vi "CreateGraphRightKeyMenu.vi"(4 "isFloatXY":T1, 6 "isShowYvalue":T1, 8 "Language":refnum<vi>, 9 "Coords":T3, 10 "MenuRef":refnum<k9>, 11 "XYGraph输入":refnum<vi>) -> ()   [LabVIEW 2015]
uses:
  <vilib>/Utility/miscctls.llb/LVPoint32TypeDef.ctl
  Ctrls/YesOrNo.ctl
panel:
  in  "WhereIsMouse":T2(ring)
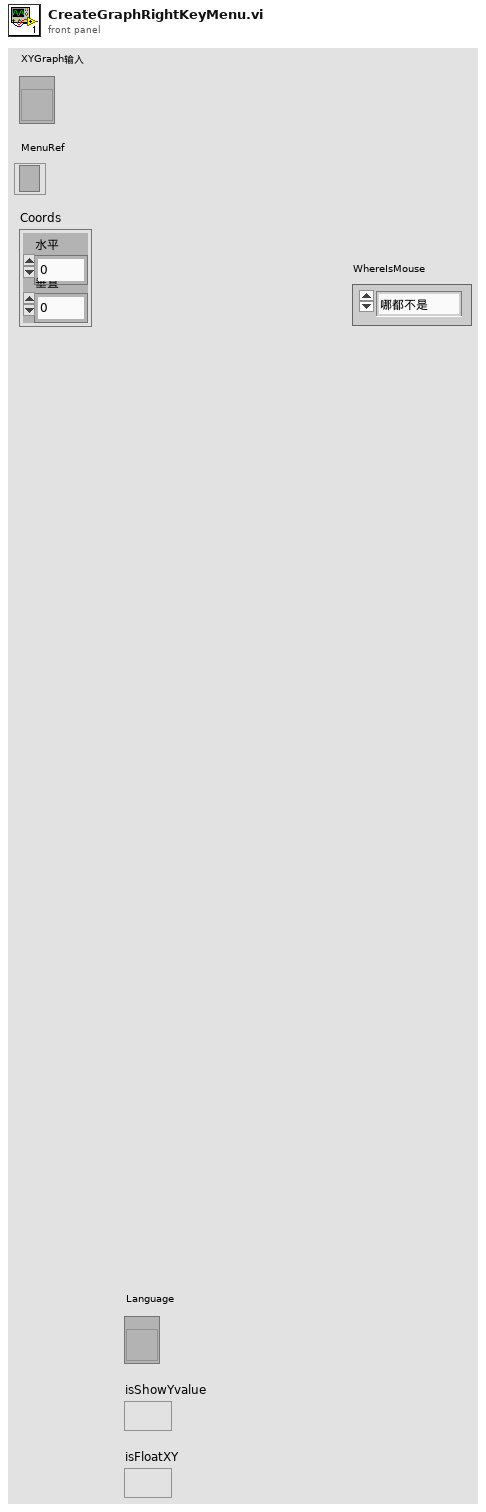
[diagram p1: front panel]
types:
  T1 = typedef "YesOrNo.ctl" = bool
  T2 = enum16{"哪都不是", "在曲线上", "在X轴上", "在单Y轴上", "在绘图区域但非曲线上", "在绘图区域上方", "在图例上"}
  T3 = typedef "LVPoint32TypeDef.ctl" = cluster{"Horizontal":i32, "Vertical":i32}
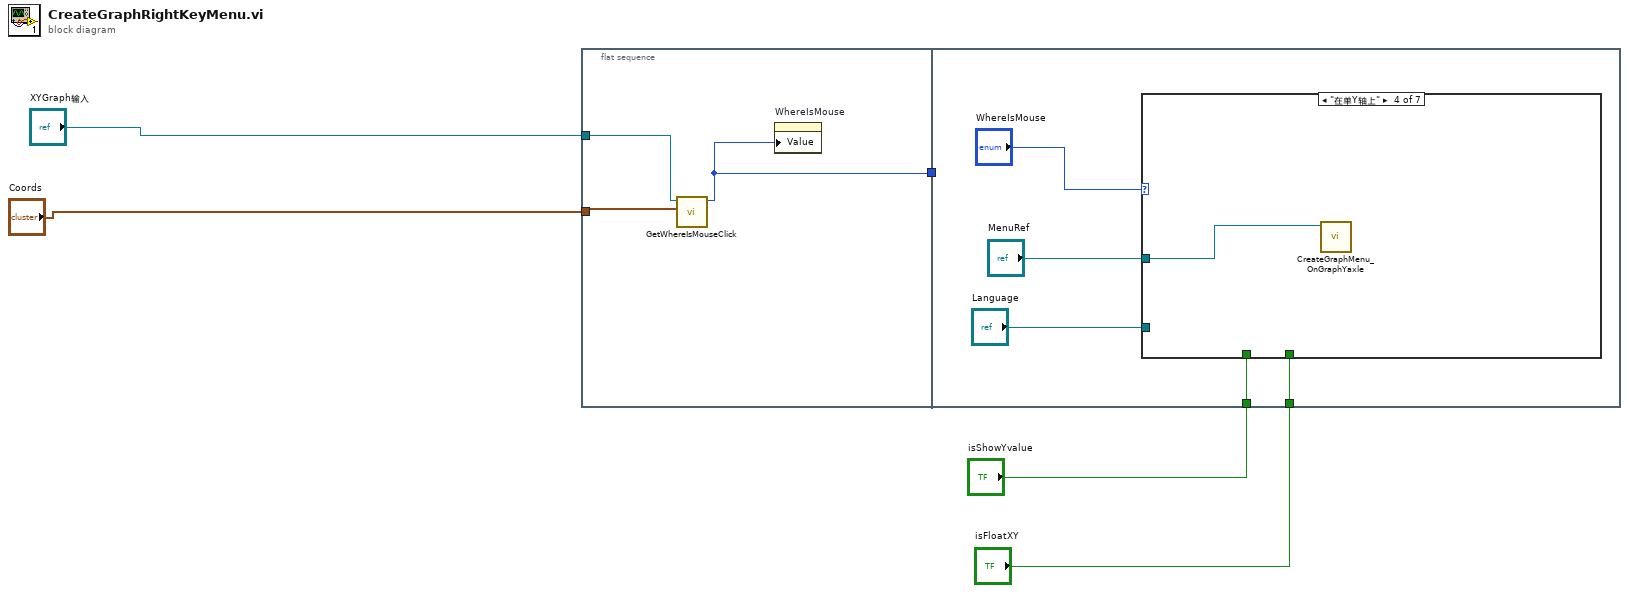
[diagram p0: block diagram]
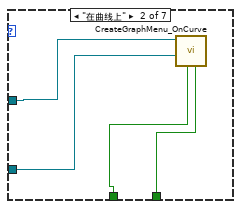
[diagram p3: hidden frame]
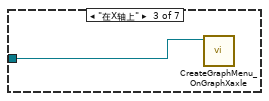
[diagram p4: hidden frame]
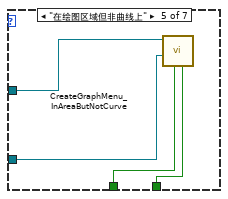
[diagram p5: hidden frame]
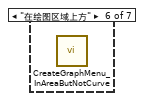
[diagram p6: hidden frame]
diagram:
  n1 = flat-sequence {
    tunnel: "XYGraph输入" -> [w8]
    tunnel: "Coords" -> [w7]
    tunnel: [w6] -> w3
    tunnel: w3 -> [_]
    tunnel: "isFloatXY" -> [w11]
    tunnel: "isShowYvalue" -> [w9]
    frame #0 {
      n2 = call "GetWhereIsMouseClick.vi"("Coords"=w7, "XYGraph输入"=w8) -> ("WhereIsMouse"=w6:T2)  [unwired: 9 in]
      n3 = property on="WhereIsMouse" class="Enum (严格)"("Value"=w6) -> ()  [unwired: 2 in, 2 out]
    }
    frame #1 {
      n4 = case shown="\"在单Y轴上\"" "WhereIsMouse" {
        tunnel: "MenuRef" -> [_ w17 w18 w19 w23 _ _]
        tunnel: w11 -> [_ w14 _ _ w20 _ _]
        tunnel: "Language" -> [_ w16 _ _ w22 _ _]
        tunnel: w9 -> [_ w15 _ _ w21 _ _]
        frame "哪都不是", Default {
        }
        frame "在曲线上" {
          n5 = call "CreateGraphMenu_OnCurve.vi"("isFloatXY"=w14, "isShowYvalue"=w15, "Language"=w16, "菜单输入"=w17) -> ()  [unwired: 8 in]
        }
        frame "在X轴上" {
          n6 = call "CreateGraphMenu_OnGraphXaxle.vi"("菜单输入"=w18) -> ()  [unwired: 11 in]
        }
        frame "在单Y轴上" {
          n7 = call "CreateGraphMenu_OnGraphYaxle.vi"("菜单输入"=w19) -> ()  [unwired: 11 in]
        }
        frame "在绘图区域但非曲线上" {
          n8 = call "CreateGraphMenu_InAreaButNotCurve.vi"("isFloatXY"=w20, "isShowYvalue"=w21, "Language"=w22, "菜单输入"=w23) -> ()  [unwired: 8 in]
        }
        frame "在绘图区域上方" {
          n9 = call "CreateGraphMenu_InAreaButNotCurve.vi"() -> ()  [unwired: 12 in]
        }
        frame "在图例上" {
        }
      }
    }
  }
